vi "Build Path Serial.vi"(8 "error in":errorcluster, 11 "Report Generator in":refnum<class "Report Generator.lvclass">) -> (0 "error out":errorcluster, 3 "Report Generator out":refnum<class "Report Generator.lvclass">)   [LabVIEW 2018, in "Report Generator.lvlib" / "Report Generator.lvclass"]
uses:
  Report Generator.lvclass
  Report Generator.lvclass/Report Generator.ctl
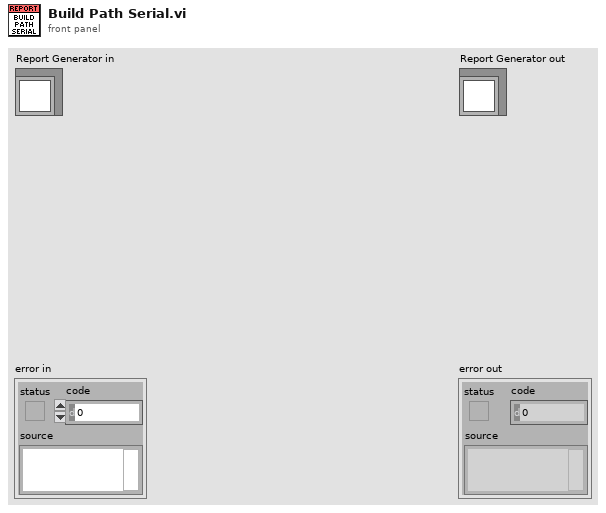
[diagram p1: front panel]
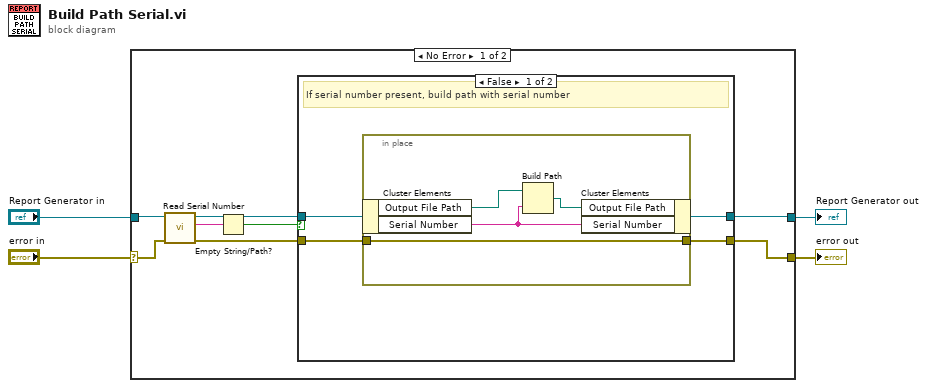
[diagram p0: block diagram]
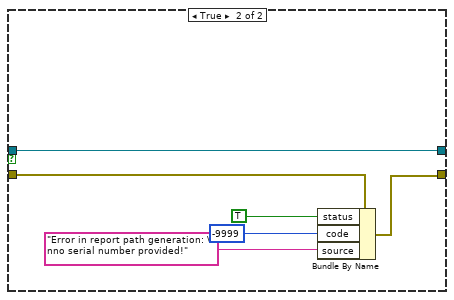
[diagram p2: hidden frame]
diagram:
  n1 = case shown="No Error" "error in" {
    selector: "error in" -> [w6 w28]
    tunnel: [w5 w28] -> w3
    tunnel: [w7 w27] -> w1
    tunnel: "Report Generator in" -> [w12 w27]
    frame No Error {
      n2 = call "Read Serial Number.vi"("error in (no error)"=w6, "Report Generator in"=w12) -> ("error out"=w8:errorcluster, "Serial Number"=w11:string, "Report Generator out"=w9:refnum<class "Report Generator.lvclass">)  [unwired: 7 in]
      n3 = Empty String/Path?(string/path=w11) -> (empty?=w10:bool)
      n4 = case shown="False" w10 {
        tunnel: w9 -> [w16 w26]
        tunnel: w8 -> [w14 w25]
        tunnel: [w15 w26] -> w7
        tunnel: [w13 w21] -> w5
        frame False {
          # "If serial number present, build path with serial number"
          n5 = in-place {
            in-place-border: w14 -> [w17]
            in-place-border: [w17] -> w13
            n6 = in-place-cluster #1(w16) -> ("Output File Path"=w20:path, "Serial Number"=w19:string)
            n7 = Build Path(base path=w20, name or relative path=w19) -> (appended path=w18:path)
            n8 = in-place-cluster #1("Output File Path"=w18, "Serial Number"=w19) -> (w15:refnum<class "Report Generator.lvclass">)
          }
        }
        frame True {
          n9 = Bundle By Name(cluster=w25, "status"=TRUE, "code"=-9999, "source"="Error in report path generation: \nno serial number provided!") -> (w21:errorcluster)
        }
      }
    }
    frame Error {
    }
  }
  "error out" <- w3
  "Report Generator out" <- w1
